vi "Zmien pozycje algorytm.vi"(8 "error in (no error)":errorcluster, 11 "Swiat in":refnum<class "Swiat.lvclass">) -> (0 "error out":errorcluster, 3 "Swiat out":refnum<class "Swiat.lvclass">)   [LabVIEW 2014, in "Swiat.lvclass"]
doc: "Generuje ruch na podstawie algorytmu przemieszczania"
uses:
  Swiat.lvclass
  Swiat.lvclass/Swiat.ctl
  Boid/Boid.lvclass/Boid.ctl
  Boid/Boid.lvclass
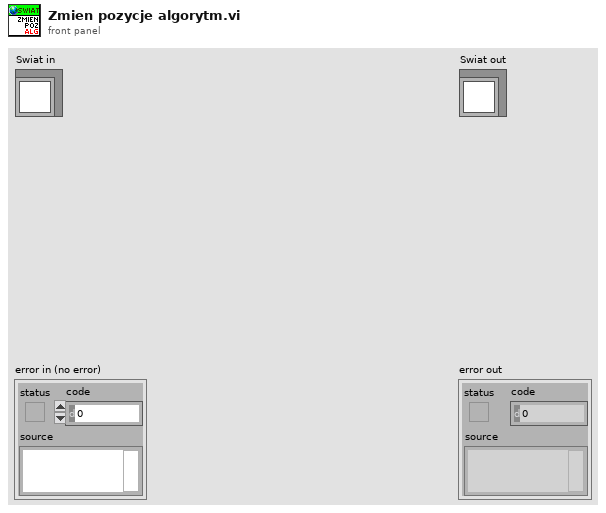
[diagram p1: front panel]
types:
  T1 = typedef "LVBoundsTypeDef.ctl" = cluster{"Width":u32, "Height":u32}
  T2 = typedef "Position.ctl" = cluster{"x":i16, "y":i16}
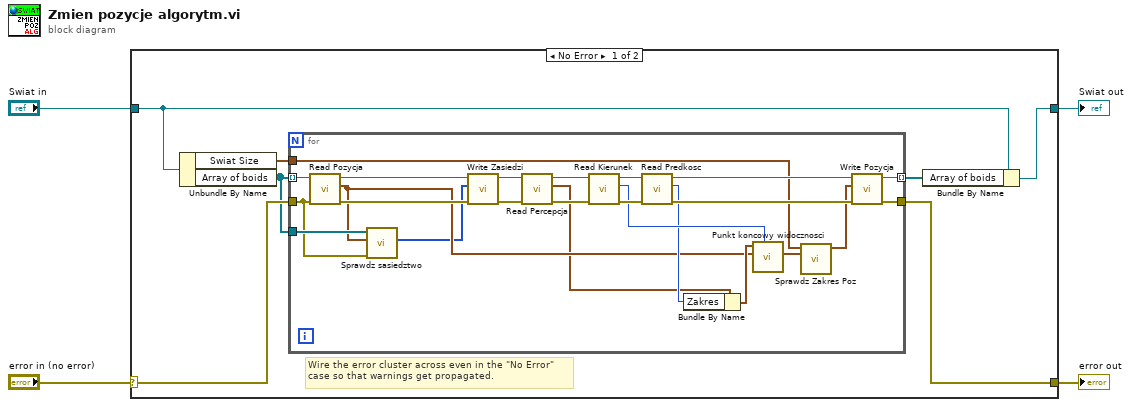
[diagram p0: block diagram]
diagram:
  n1 = case shown="No Error" "error in (no error)" {
    selector: "error in (no error)" -> [w8 w36]
    tunnel: [w7 w36] -> w1
    tunnel: [w10 w37] -> w2
    tunnel: "Swiat in" -> [w11 w37]
    frame No Error {
      # "Wire the error cluster across even in the \"No Error\"\ncase so that warnings get propagated."
      n2 = Unbundle By Name(w11) -> ("Swiat Size"=w6:T1, "Array of boids"=w5:refnum<class "Boid.lvclass">[])
      n3 = for {
        tunnel: w5 -> [w23] mode=indexing
        tunnel: w8 -> [w19]
        tunnel: [w31] -> w9 mode=indexing
        tunnel: [w30] -> w7
        tunnel: w6 -> [w24]
        tunnel: w5 -> [w20]
        n4 = call "Read Pozycja.vi"("error in (no error)"=w19, "Boid in"=w23) -> ("error out"=w21:errorcluster, "Position"=w18:T2, "Boid out"=w22:refnum<class "Boid.lvclass">)  [unwired: 7 in]
        n5 = call "Sprawdz sasiedztwo.vi"("error in (no error)"=w19, "Position"=w18, "Array of boids"=w20) -> ("Sasiedzi"=w17:i32[])  [unwired: 8 in]
        n6 = call "Write Zasiedzi.vi"("error in (no error)"=w21, "Zasiedzi"=w17, "Boid in"=w22) -> ("error out"=w16:errorcluster, "Boid out"=w15:refnum<class "Boid.lvclass">)  [unwired: 7 in]
        n7 = call "Read Percepcja.vi"("error in (no error)"=w16, "Boid in"=w15) -> ("error out"=w13:errorcluster, "Percepcja"=w12:cluster{"Zakres":i16, "Kat":i16}, "Boid out"=w14:refnum<class "Boid.lvclass">)  [unwired: 7 in]
        n8 = call "Read Kierunek.vi"("error in (no error)"=w13, "Boid in"=w14) -> ("error out"=w35:errorcluster, "Kierunek"=w29:i16, "Boid out"=w34:refnum<class "Boid.lvclass">)  [unwired: 7 in]
        n9 = call "Read Predkosc.vi"("error in (no error)"=w35, "Boid in"=w34) -> ("error out"=w32:errorcluster, "Predkosc"=w27:i16, "Boid out"=w33:refnum<class "Boid.lvclass">)  [unwired: 7 in]
        n10 = Bundle By Name(cluster=w12, "Zakres"=w27) -> (w28:cluster{"Zakres":i16, "Kat":i16})
        n11 = call "Punkt koncowy widocznosci.vi"("Kierunek"=w29, "Start Pos"=w18, "Percepcja"=w28) -> ("Final Pos"=w26:T2)  [unwired: 7 in, 1 out]
        n12 = call "Sprawdz Zakres Poz.vi"("Pos in"=w26, "Swiat Size"=w24) -> ("Pos out"=w25:T2)  [unwired: 8 in, 1 out]
        n13 = call "Write Pozycja.vi"("error in (no error)"=w32, "Position"=w25, "Boid in"=w33) -> ("error out"=w30:errorcluster, "Boid out"=w31:refnum<class "Boid.lvclass">)  [unwired: 7 in]
      }
      n14 = Bundle By Name(cluster=w11, "Array of boids"=w9) -> (w10:refnum<class "Swiat.lvclass">)
    }
    frame Error {
    }
  }
  "error out" <- w1
  "Swiat out" <- w2
